vi "Do Core.vi"(8 "error in (no error)":errorcluster, 9 "Actor in":refnum<class "Actor.lvclass">, 11 "Divide Msg.lvclass":refnum<class "Divide Msg.lvclass">) -> (0 "error out":errorcluster, 1 "Actor out":refnum<class "Actor.lvclass">, 2 "Variant":variant)   [LabVIEW 2012, in "Divide Msg.lvclass"]
uses:
  Divide Msg.lvclass
  <vilib>/ActorFramework/Actor/Actor.lvclass
  TestActor/TestActor.lvclass
  Increment2 Msg/Increment2 Msg.lvclass
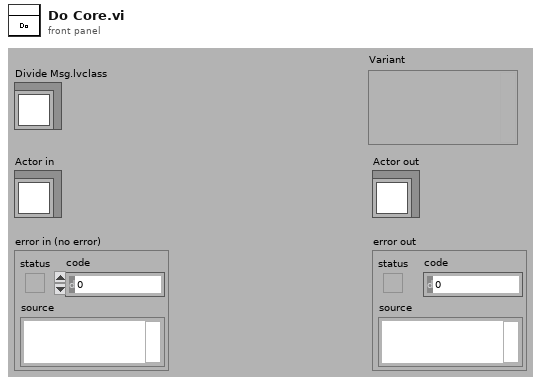
[diagram p1: front panel]
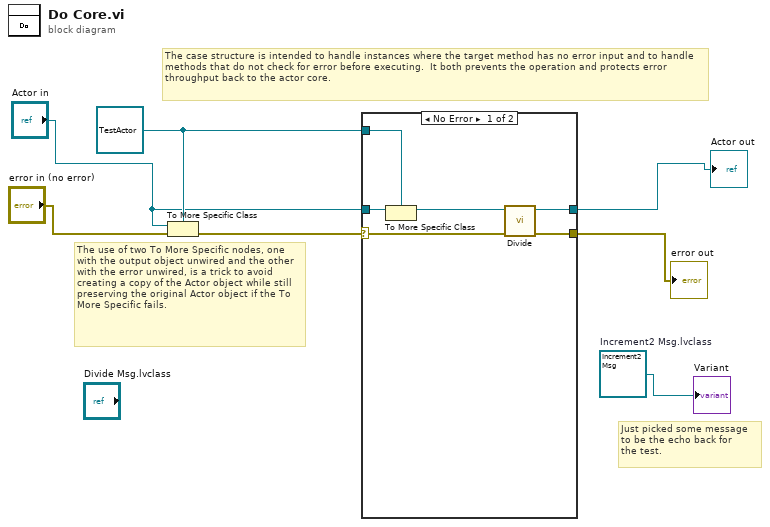
[diagram p0: block diagram]
diagram:
  w1 = refnum<class "Increment2 Msg.lvclass"> refnum  # Increment2 Msg.lvclass
  w6 = refnum<class "TestActor.lvclass"> refnum ("Actor in")
  # "Just picked some message\nto be the echo back for\nthe test."
  # "The use of two To More Specific nodes, one with the output object unwired and the other with the error unwired, is a trick to avoid creating a copy of the Actor object while still preserving the original Actor object if the To More Specific fails."
  # "The case structure is intended to handle instances where the target method has no error input and to handle methods that do not check for error before executing.  It both prevents the operation and protects error throughput back to the actor core."
  n1 = To More Specific Class(target class=w6, reference="Actor in", error in="error in (no error)") -> (error out=w7:errorcluster)  [unwired: 1 out]
  n2 = case shown="No Error" w7 {
    selector: w7 -> [w11 w15]
    tunnel: [w13 w15] -> w2
    tunnel: [w12 w14] -> w3
    tunnel: "Actor in" -> [w10 w14]
    tunnel: w6 -> [w9 _]
    frame No Error {
      n3 = To More Specific Class(target class=w9, reference=w10) -> (specific class reference=w8:refnum<class "TestActor.lvclass">)  [unwired: 1 in, 1 out]
      n4 = call "Divide.vi"("error in (no error)"=w11, "TestActor in"=w8) -> ("error out"=w13:errorcluster, "TestActor out"=w12:refnum<class "TestActor.lvclass">)  [unwired: 8 in]
    }
    frame Error {
      # "If type check fails, pass the original object out again."
    }
  }
  "Actor out" <- w3
  "error out" <- w2
  "Variant" <- w1
